vi "8.7.-Momento h4.vi"(1 "n30/n12/n21/n03":dbl[](array[numeric])) -> (0 "M4":dbl)   [LabVIEW 2020]
panel:
  # "Visión Artificial - Momentos Invariantes de Hu\nDiego Cervantes Rodríguez\ndicer0.com"
  # "M4 = ((n30+n12)^2)+((n21+n03)^2)"
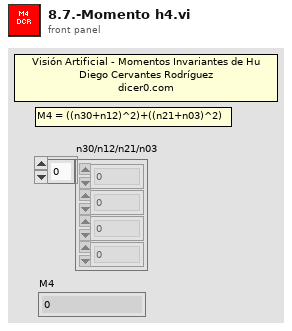
[diagram p1: front panel]
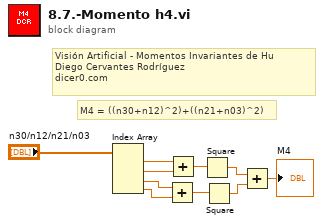
[diagram p0: block diagram]
diagram:
  # "Visión Artificial - Momentos Invariantes de Hu\nDiego Cervantes Rodríguez\ndicer0.com"
  # "M4 = ((n30+n12)^2)+((n21+n03)^2)"
  n1 = Index Array "Index Array"(array="n30/n12/n21/n03") -> (element #1=w9:dbl, element #2=w8:dbl, element #3=w7:dbl, element #4=w6:dbl)  [unwired: 4 in]
  n2 = Add(x=w7, y=w6) -> (x+y=w4:dbl)
  n3 = Add(x=w9, y=w8) -> (x+y=w5:dbl)
  n4 = Square(x=w5) -> (x^2=w3:dbl)
  n5 = Square(x=w4) -> (x^2=w2:dbl)
  n6 = Add(x=w3, y=w2) -> (x+y=→"M4":dbl)
